vi "Get Minimum Image Length.vi"(11 "MinImageLength":i32) -> (2 "function return":u32, 3 "MinImageLength out":i32)   [LabVIEW 2018, in "AndorSDK.lvlib"]
doc: "EXPNETTYPE unsigned int WINAPI GetMinimumImageLength(int * MinImageLength);"
uses:
  AndorSDK.lvlib
  ATMCD32D.dll
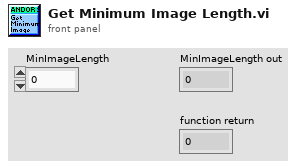
[diagram p1: front panel]
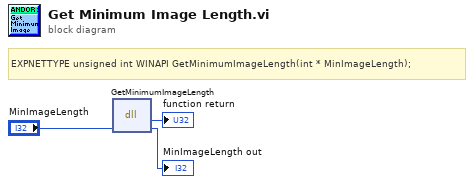
[diagram p0: block diagram]
diagram:
  # "EXPNETTYPE unsigned int WINAPI GetMinimumImageLength(int * MinImageLength);"
  n1 = dll-call lib="PTH2babs E\nPersönliches02 - Arbeit03-HiwijobsLabviewCodelibANDOR\tAndor SDK\nATMCD32D.*" fn="GetMinimumImageLength"("MinImageLength"="MinImageLength") -> (→"function return":u32, "MinImageLength"=→"MinImageLength out":i32)  [unwired: 3 in, 2 out]
